vi "Test_AI_AO_v7_HighSampleRate.vi"() -> ()   [LabVIEW 2017]
uses:
  <vilib>/DAQmx/read.llb/DAQmx Read (Analog 1D Wfm NChan 1Samp).vi
  <vilib>/DAQmx/write.llb/DAQmx Write (Analog DBL 1Chan 1Samp).vi
  <vilib>/DAQmx/write.llb/DAQmx Write (Digital Wfm 1Chan NSamp).vi
  <vilib>/DAQmx/create/channels.llb/DAQmx Create Channel (AO-Voltage-Basic).vi
  <vilib>/DAQmx/create/channels.llb/DAQmx Create Channel (AI-Voltage-Basic).vi
  <vilib>/DAQmx/create/channels.llb/DAQmx Create Channel (DO-Digital Output).vi
  <vilib>/DAQmx/miscellaneous.llb/DAQmx Fill In Error Info.vi
  <vilib>/Waveform/DWDTOps.llb/DWDT Analog to Digital.vi
  <vilib>/Waveform/DWDTOps.llb/DWDT Uncompress Digital.vi
  <vilib>/DAQmx/configure/timing.llb/DAQmx Timing (Sample Clock).vi
  <vilib>/measure/NI_MABase.lvlib
panel:
  in  "Driving Current\nAmplitude (mA)":dbl=500.0 format="%0.2f"
  in  "time for Presenting Pattern":u32=1000
  in  "Sample rate":dbl=1000.0 format="%0.2f"
  out "Measurement 6":waveform(dbl)(graph)={"t0"=timestamp(3694524964.9017587 s since 1904-01-01), "dt"=0.001, "Y"=[-0.02074009728149634], "attributes"=variant("NI_ChannelName"=variant(string "Dev1/ai4"), "NI_UnitDescription"=variant(string "Volts"))} caption="Optometer"
  in  "lines":tag="Dev1/port1/line1"
  in  "Combo Box":string(combo)="Huge LED"
  out "File name":string="Test_210127015551.csv"
  in  "file path (use dialog)":path=path "C:/Users/Fukunaga/Documents/Xiaochen/Code/DMD_ephys/Folder Test/Trigger_DMD"
  out "Measurement 5":waveform(dbl)(graph)={"t0"=timestamp(3694524964.9017587 s since 1904-01-01), "dt"=0.001, "Y"=[3.323040226828381], "attributes"=variant("NI_ChannelName"=variant(string "Dev1/ai7"), "NI_UnitDescription"=variant(string "Volts"))} caption="Trigger 2"
  out "Measurement 3":waveform(dbl)(graph)={"t0"=timestamp(3694524964.9017587 s since 1904-01-01), "dt"=0.001, "Y"=[0.019601763716835273], "attributes"=variant("NI_ChannelName"=variant(string "Dev1/ai6"), "NI_UnitDescription"=variant(string "Volts"))} caption="Trigger 1"
  in  "AO Illumination":tag="Dev1/ao0"
  in  "time for uploading":u32=2000
  out "Measurement 2":waveform(dbl)(graph)={"t0"=timestamp(0 s since 1904-01-01), "dt"=0.001, "Y"=[1.0, 1.0, 1.0, 1.0, 1.0, 1.0, 1.0, 1.0, 1.0, 1.0, 1.0, 1.0, 1.0, 1.0, 1.0, 1.0, 1.0, 1.0, 1.0, 1.0, 1.0, 1.0, 1.0, 1.0, 1.0, 1.0, 1.0, 1.0, 1.0, 1.0, 0.0, 0.0, 0.0, 0.0, 0.0, 0.0, 0.0, 0.0, 0.0, 0.0, 0.0, 0.0, 0.0, 0.0, 0.0, 0.0, 0.0, 0.0, 0.0, 0.0, 0.0, 0.0, 0.0, 0.0, 0.0, 0.0, 0.0, 0.0, 0.0, 0.0, 0.0, 0.0, 0.0, 0.0, 0.0, 0.0, 0.0, 0.0, 0.0, 0.0, 0.0, 0.0, 0.0, 0.0, 0.0, 0.0, 0.0, 0.0, 0.0, 0.0, 0.0, 0.0, 0.0, 0.0, 0.0, 0.0, 0.0, 0.0, 0.0, 0.0, 0.0, 0.0, 0.0, 0.0, 0.0, 0.0, 0.0, 0.0, 0.0, 0.0]} caption="output"
  in  "Number of Pulse":i8=1
  in  "DMD Pulse \nDuration (ms)":dbl=30.0
  in  "timeout":dbl=0.1 format="%0.2f"
  in  "Frequency of Pulse (Hz)":dbl=10.0
  in  "amplitude":dbl=1.0
  in  "AO UploadDMD":tag="Dev1/ao1"
  in  "Stop Sampling":bool
  in  "latency between two stimuli":u32=1000
  in  "Stop Stimuli":bool
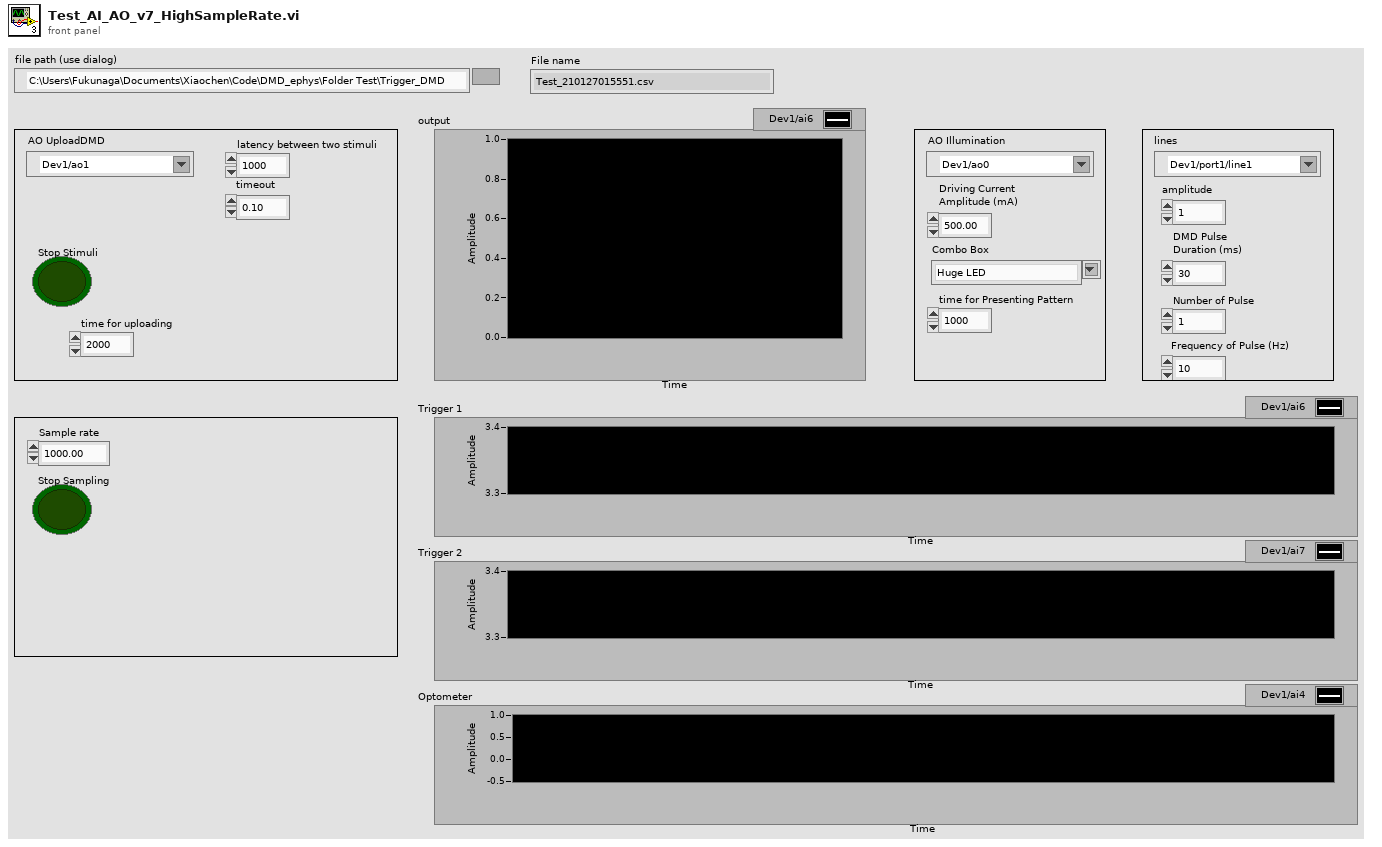
[diagram p1: front panel]
types:
  T1 = enum16{"open", "replace", "create", "open or create", "replace or create", "replace or create with confirmation"}
  T2 = enum16{"Sine Wave", "Triangle Wave", "Square Wave", "Sawtooth Wave"}
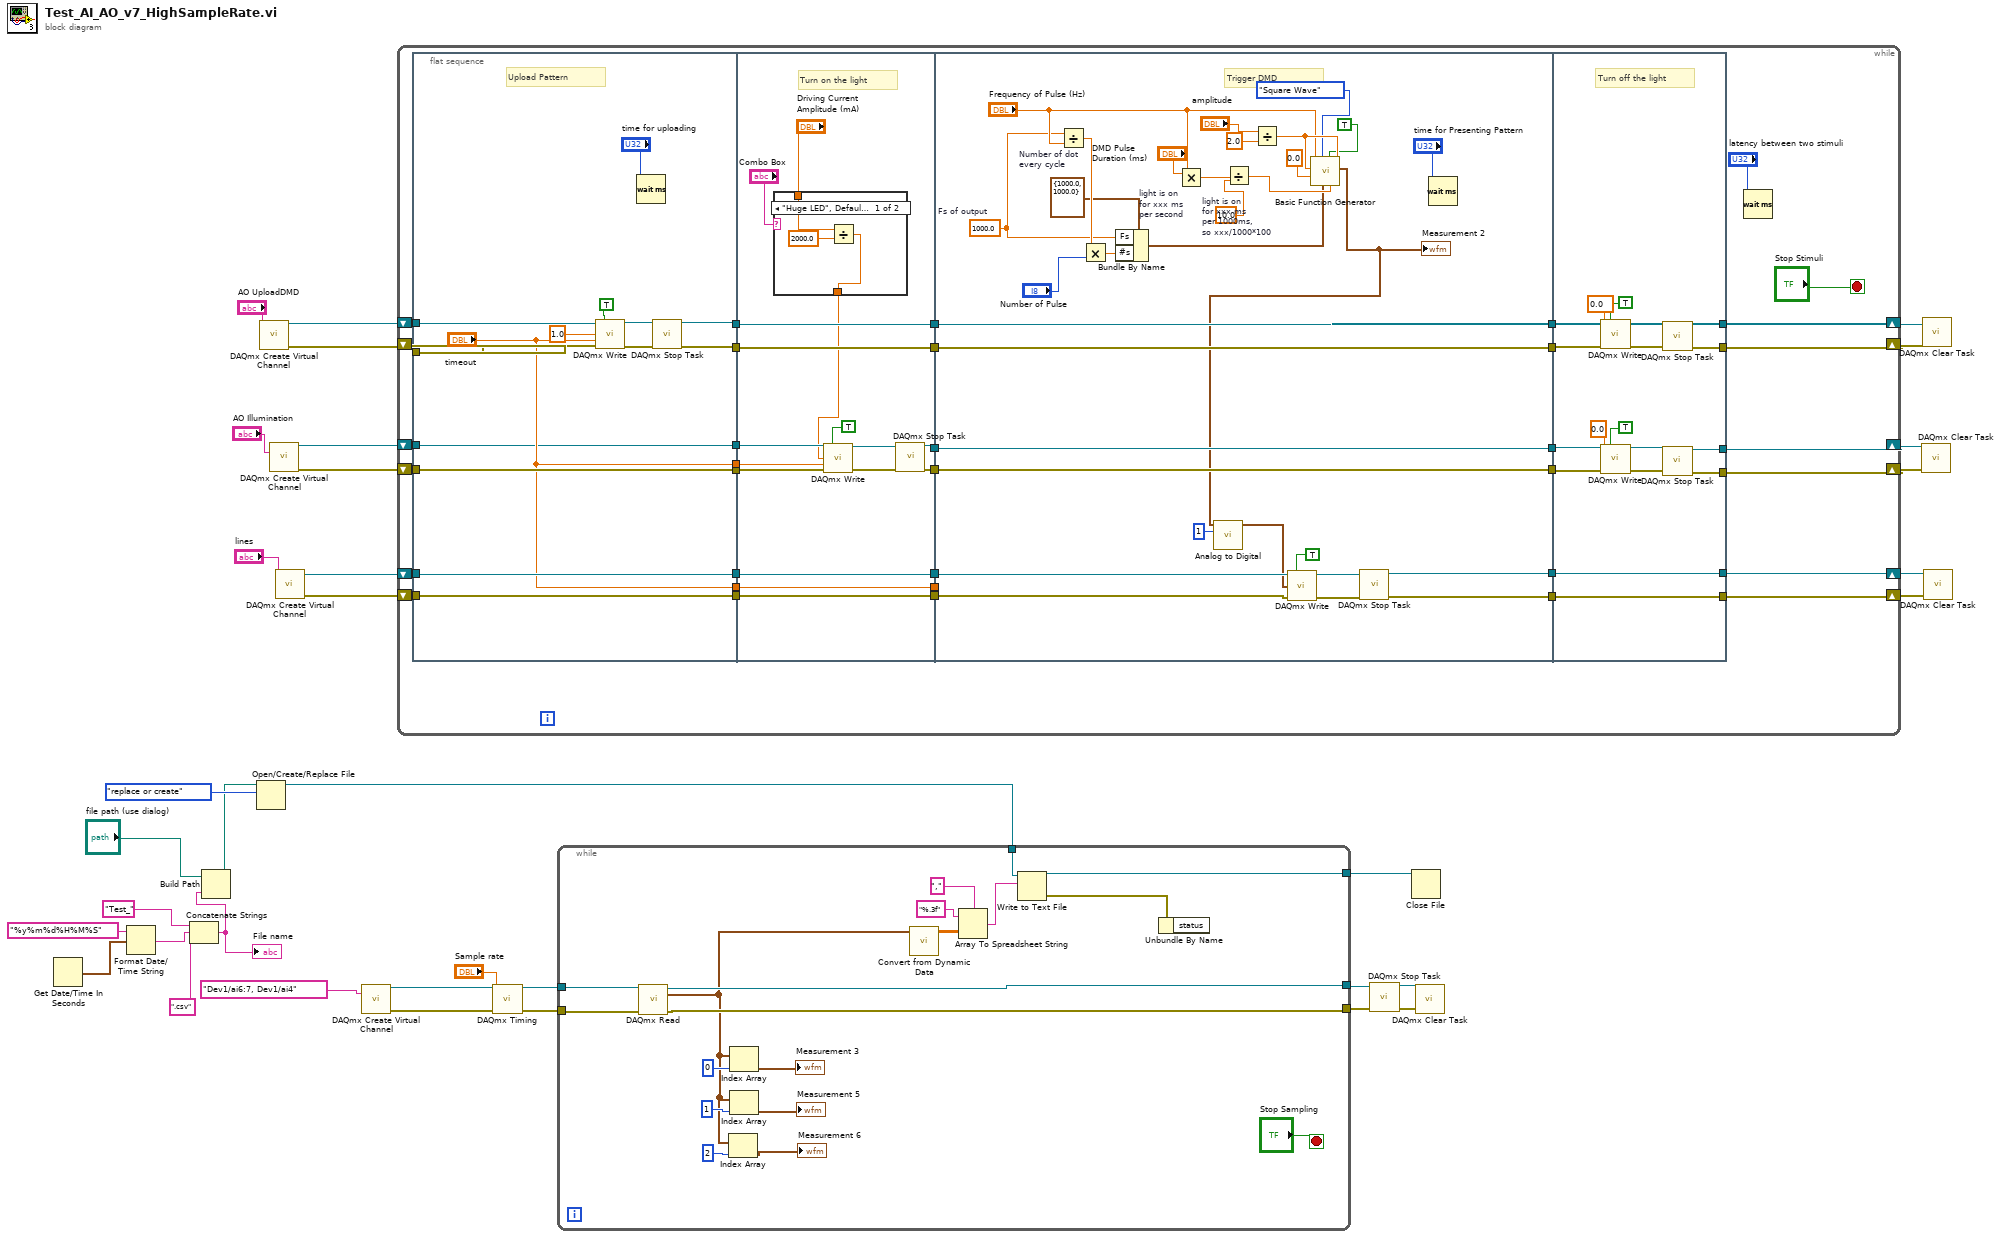
[diagram p0: block diagram]
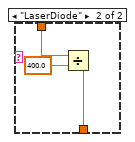
[diagram p2: hidden frame]
diagram:
  n1 = Get Date/Time In Seconds() -> (seconds since 1Jan1904=w20:timestamp)
  n2 = Format Date/Time String(time format string (%c)="%y%m%d%H%M%S", seconds (now)=w20) -> (date/time string=w17:string)  [unwired: 1 in]
  n3 = Concatenate Strings("Test_" ("string"), w17, ".csv" ("string")) -> (w15:string)
  "File name" <- w15
  n4 = Build Path(base path="file path (use dialog)", name or relative path=w15) -> (appended path=w18:path)
  n5 = Open/Create/Replace File(file path (use dialog)=w18, operation (0:open)=T1."replace or create") -> (refnum out=w12:refnum<file>)  [unwired: 4 in, 2 out]
  n6 = call-poly <vilib>:"DAQmx Create Virtual Channel.vi"("physical channels"="AO UploadDMD") -> ("task out"=w35:refnum<k21>, "error out"=w33:errorcluster)  [unwired: 13 in]
  n7 = call-poly <vilib>:"DAQmx Create Virtual Channel.vi"("physical channels"="AO Illumination") -> ("task out"=w29:refnum<k21>, "error out"=w31:errorcluster)  [unwired: 13 in]
  n8 = call-poly <vilib>:"DAQmx Create Virtual Channel.vi"("lines"="lines") -> ("task out"=w10:refnum<k21>, "error out"=w11:errorcluster)  [unwired: 13 in]
  n9 = call-poly <vilib>:"DAQmx Create Virtual Channel.vi"("physical channels"=tag "Dev1/ai6:7, Dev1/ai4" ("Input channel 1")) -> ("task out"=w3:refnum<k21>, "error out"=w4:errorcluster)  [unwired: 13 in]
  n10 = while {
    shift-right: [w69] -> w34
    shift-left: w35 -> [w70]
    shift-right: [w67] -> w32
    shift-left: w33 -> [w68]
    shift-right: [w50] -> w30
    shift-left: w31 -> [w63]
    shift-right: [w49] -> w8
    shift-left: w29 -> [w61]
    shift-right: [w44] -> w7
    shift-left: w10 -> [w48]
    shift-right: [w42] -> w9
    shift-left: w11 -> [w39]
    stop <- "Stop Stimuli" stop-if-true
    n11 = flat-sequence {
      tunnel: w70 -> [w82]
      tunnel: w68 -> [w80]
      tunnel: [w81] -> w66
      tunnel: [w79] -> w65
      tunnel: w63 -> [w78]
      tunnel: [w78] -> w62
      tunnel: w61 -> [w73]
      tunnel: [w73] -> w60
      tunnel: ["timeout"] -> w59
      tunnel: w48 -> [w77]
      tunnel: [w77] -> w47
      tunnel: [w76] -> w40
      tunnel: w39 -> [w76]
      tunnel: ["timeout"] -> w38
      tunnel: w66 -> [w100]
      tunnel: w65 -> [w99]
      tunnel: w62 -> [w97]
      tunnel: w60 -> [w94]
      tunnel: w59 -> [w93]
      tunnel: [w100] -> w58
      tunnel: [w99] -> w57
      tunnel: [w97] -> w56
      tunnel: [w95] -> w55
      tunnel: w47 -> [w91]
      tunnel: [w91] -> w46
      tunnel: [w90] -> w41
      tunnel: w40 -> [w90]
      tunnel: w38 -> [w89]
      tunnel: [w89] -> w37
      tunnel: w58 -> [w138]
      tunnel: w57 -> [w137]
      tunnel: w56 -> [w136]
      tunnel: w55 -> [w135]
      tunnel: [w138] -> w54
      tunnel: [w137] -> w53
      tunnel: [w136] -> w52
      tunnel: [w135] -> w51
      tunnel: w46 -> [w131]
      tunnel: [w130] -> w45
      tunnel: [w129] -> w43
      tunnel: w41 -> [w128]
      tunnel: w37 -> [_]
      tunnel: [w139] -> w67
      tunnel: [w140] -> w69
      tunnel: w54 -> [w142]
      tunnel: w53 -> [w141]
      tunnel: w52 -> [w149]
      tunnel: w51 -> [w150]
      tunnel: [w152] -> w50
      tunnel: [w151] -> w49
      tunnel: w45 -> [w148]
      tunnel: [w148] -> w44
      tunnel: w43 -> [w147]
      tunnel: [w147] -> w42
      frame #0 {
        # "Upload Pattern"
        n12 = call-poly <vilib>:"DAQmx Write.vi"("task/channels in"=w82, "auto start"=TRUE, "data"=1.0, "timeout"="timeout", "error in"=w80) -> ("task out"=w84:refnum<k21>, "error out"=w83:errorcluster)  [unwired: 8 in, 1 out]
        n13 = Wait (ms)(milliseconds to wait="time for uploading") -> ()  [unwired: 1 out]
        n14 = call <vilib>:"DAQmx Stop Task.vi"("task/channels in"=w84, "error in"=w83) -> ("task out"=w81:refnum<k21>, "error out"=w79:errorcluster)  [unwired: 12 in]
      }
      frame #1 {
        # "Turn on the light"
        n15 = case shown="\"Huge LED\", Default" "Combo Box" {
          tunnel: "Driving Current\nAmplitude (mA)" -> [w103 w106]
          tunnel: [w101 w104] -> w87
          frame "Huge LED", Default {
            n16 = Divide(x=w103, y=2000.0) -> (x/y=w101:dbl)
          }
          frame "LaserDiode" {
            n17 = Divide(x=w106, y=400.0) -> (x/y=w104:dbl)
          }
        }
        n18 = call-poly <vilib>:"DAQmx Write.vi"("task/channels in"=w94, "auto start"=TRUE, "data"=w87, "timeout"=w93, "error in"=w97) -> ("task out"=w96:refnum<k21>, "error out"=w98:errorcluster)  [unwired: 8 in, 1 out]
        n19 = call <vilib>:"DAQmx Stop Task.vi"("task/channels in"=w96, "error in"=w98) -> ("task out"=w95:refnum<k21>)  [unwired: 12 in, 1 out]
      }
      frame #2 {
        w115 = 1000.0  # Fs of output
        # "Trigger DMD"
        n20 = Divide "Number of dot \nevery cycle"(x=w115, y="Frequency of Pulse (Hz)") -> (x/y=w120:dbl)
        n21 = Multiply(x=w120, y="Number of Pulse") -> (x*y=w124:dbl)
        n22 = Bundle By Name(cluster=cluster{"Fs":dbl, "#s":dbl} {"Fs"=1000.0, "#s"=1000.0} ("sampling info"), "Fs"=w115, "#s"=w124) -> (w118:cluster{"Fs":dbl, "#s":dbl})
        n23 = Multiply "light is on \nfor xxx ms \nper second"(x="DMD Pulse \nDuration (ms)", y="Frequency of Pulse (Hz)") -> (x*y=w123:dbl)
        n24 = Divide "light is on \nfor xxx ms \nper 1000ms,\nso xxx/1000*100"(x=w123, y=10.0) -> (x/y=w125:dbl)
        n25 = Divide(x="amplitude", y=2.0) -> (x/y=w127:dbl)
        n26 = call <vilib>:"Basic Function Generator.vi"("offset"=w127, "square wave duty cycle (%)"=w125, "reset signal"=TRUE, "sampling info"=w118, "signal type"=T2."Square Wave", "phase"=0.0, "amplitude"=w127, "frequency"="Frequency of Pulse (Hz)") -> ("signal out"=w110:waveform(dbl))  [unwired: 1 in, 2 out]
        "Measurement 2" <- w110
        n27 = call-poly <vilib>:"Analog to Digital.vi"("resolution (16 bit)"=1, "analog waveform"=w110) -> ("digital waveform"=w109:digitalwaveform)  [unwired: 6 in, 3 out]
        n28 = call-poly <vilib>:"DAQmx Write.vi"("task/channels in"=w131, "auto start"=TRUE, "data"=w109, "error in"=w128) -> ("task out"=w133:refnum<k21>, "error out"=w134:errorcluster)  [unwired: 9 in, 1 out]
        n29 = call <vilib>:"DAQmx Stop Task.vi"("task/channels in"=w133, "error in"=w134) -> ("task out"=w130:refnum<k21>, "error out"=w129:errorcluster)  [unwired: 12 in]
        n30 = Wait (ms)(milliseconds to wait="time for Presenting Pattern") -> ()  [unwired: 1 out]
      }
      frame #3 {
        # "Turn off the light"
        n31 = call-poly <vilib>:"DAQmx Write.vi"("task/channels in"=w142, "auto start"=TRUE, "data"=0.0 ("data 2"), "error in"=w141) -> ("task out"=w145:refnum<k21>, "error out"=w146:errorcluster)  [unwired: 9 in, 1 out]
        n32 = call-poly <vilib>:"DAQmx Write.vi"("task/channels in"=w150, "auto start"=TRUE, "data"=0.0 ("data 2"), "error in"=w149) -> ("task out"=w155:refnum<k21>, "error out"=w156:errorcluster)  [unwired: 9 in, 1 out]
        n33 = call <vilib>:"DAQmx Stop Task.vi"("task/channels in"=w145, "error in"=w146) -> ("task out"=w140:refnum<k21>, "error out"=w139:errorcluster)  [unwired: 12 in]
        n34 = call <vilib>:"DAQmx Stop Task.vi"("task/channels in"=w155, "error in"=w156) -> ("task out"=w151:refnum<k21>, "error out"=w152:errorcluster)  [unwired: 12 in]
      }
    }
    n35 = Wait (ms)(milliseconds to wait="latency between two stimuli") -> ()  [unwired: 1 out]
  }
  n36 = call-poly <vilib>:"DAQmx Timing.vi"("task/channels in"=w3, "rate"="Sample rate", "error in"=w4) -> ("task out"=w2:refnum<k21>, "error out"=w5:errorcluster)  [unwired: 11 in]
  n37 = while {
    tunnel: w2 -> [w174]
    tunnel: w5 -> [w173]
    tunnel: [w172] -> w26
    tunnel: [w171] -> w25
    tunnel: [w161] -> w13
    tunnel: w12 -> [w160]
    stop <- "Stop Sampling" stop-if-true
    n38 = call-poly <vilib>:"DAQmx Read.vi"("task/channels in"=w174, "error in"=w173) -> ("task out"=w172:refnum<k21>, "data"=w157:waveform(dbl)[], "error out"=w171:errorcluster)  [unwired: 11 in]
    n39 = Index Array(array=w157, index=2) -> (element=→"Measurement 6":waveform(dbl))
    n40 = Index Array(array=w157, index=0) -> (element=→"Measurement 3":waveform(dbl))
    n41 = Index Array(array=w157, index=1) -> (element=→"Measurement 5":waveform(dbl))
    n42 = call "Convert from Dynamic Data"("Dynamic Data Type"=w157) -> ("Array"=w162:dbl[][])  [unwired: 3 in]
    n43 = Array To Spreadsheet String(delimiter (Tab)=",", array=w162, 3:"%.3f" ("format string")) -> (spreadsheet string=w163:string)
    n44 = Write to Text File(file (use dialog)=w160, text=w163) -> (refnum out=w161:refnum<file>, error out=w166:errorcluster)  [unwired: 2 in, 1 out]
    n45 = Unbundle By Name(w166) -> ()  [unwired: 1 out]
  }
  n46 = call <vilib>:"DAQmx Stop Task.vi"("task/channels in"=w26, "error in"=w25) -> ("task out"=w24:refnum<k21>, "error out"=w23:errorcluster)  [unwired: 12 in]
  n47 = Close File(refnum=w13) -> ()  [unwired: 1 in, 2 out]
  n48 = call <vilib>:"DAQmx Clear Task.vi"("task in"=w24, "error in"=w23) -> ()  [unwired: 13 in, 1 out]
  n49 = call <vilib>:"DAQmx Clear Task.vi"("task in"=w8, "error in"=w30) -> ()  [unwired: 13 in, 1 out]
  n50 = call <vilib>:"DAQmx Clear Task.vi"("task in"=w34, "error in"=w32) -> ()  [unwired: 13 in, 1 out]
  n51 = call <vilib>:"DAQmx Clear Task.vi"("task in"=w7, "error in"=w9) -> ()  [unwired: 13 in, 1 out]
